vi "HEWH Check NA Skip Conditions.vi"(8 "Error In":errorcluster, 11 "Current Input":T1) -> (0 "Error Out":errorcluster, 3 "N/A or Skip?":bool)   [LabVIEW 2020]
uses:
  Type Definitions/HEWH Special Condition Check.ctl
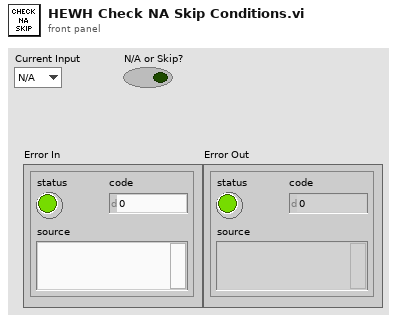
[diagram p1: front panel]
types:
  T1 = typedef "HEWH Special Condition Check.ctl" = enum16{"N/A", "C1", "C2", "Reset/Fail", "Skip Draw Sequence"}
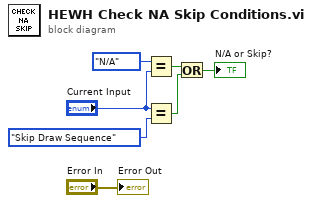
[diagram p0: block diagram]
diagram:
  n1 = Equal?(x=HEWH_Special_Condition_Check."N/A" ("y"), y="Current Input") -> (x = y?=w4:bool)
  n2 = Equal?(x="Current Input", y=HEWH_Special_Condition_Check."Skip Draw Sequence") -> (x = y?=w5:bool)
  n3 = Or(x=w4, y=w5) -> (x .or. y?=→"N/A or Skip?":bool)
  "Error Out" <- "Error In"
